vi "pid-waterController.vi"() -> ()   [LabVIEW 2011]
uses:
  <vilib>/Simulation/Scripting/Companion Diagram/SimConfigNode/SimParams.ctl
  <vilib>/Simulation/Scripting/Companion Diagram/SimConfigNode/_simSolvers.ctl
  <vilib>/Simulation/Implementation/Shared/SIMSCR Execution Mode.ctl
  <vilib>/Simulation/Param Hierarchy/Typedefs/SIMPH Param Control Actions.ctl
  <vilib>/Simulation/Implementation/Shared/NILVSim_FinalizeModel.vi
  <vilib>/Simulation/Implementation/Shared/NILVSim_Manager.vi
  <vilib>/Simulation/Implementation/Shared/NILVSim_ParamChanged.vi
  <vilib>/MakerHub/LINX/Public/Peripherals/PWM/PWM Set Duty Cycle 1 Chan.vi
  <vilib>/MakerHub/LINX/Public/Utilities/Open Serial.vi
  <vilib>/Simulation/Implementation/Shared/SIM Unbundle Sim Info.vi
  <vilib>/Simulation/Implementation/Shared/NILVSim_GetModelError.vi
  <vilib>/Simulation/Implementation/Shared/SIM Bundle Sim Info.vi
  <vilib>/Simulation/Implementation/Shared/NILVSim_Initialize.vi
  <vilib>/MakerHub/LINX/Public/Peripherals/PWM/PWM Set Duty Cycle N Chans.vi
  <vilib>/Simulation/Implementation/XNodeFramework/SimXNode/SimX.xnode
  <vilib>/Simulation/Model Libraries/PID/SIM PID (Academic).vi
  <vilib>/Simulation/Model Libraries/PID/SIM PID.vi
  <vilib>/Simulation/Scripting/Companion Diagram/SimConfigNode/SimDog.xnode
  <vilib>/MakerHub/LINX/LMH-LINX.lvlib
  <vilib>/Simulation/Implementation/Shared/NI_SIM_Implementation.lvlib
panel:
  out "PID Output":dbl
  out "Tank":dbl(slide) scale=0.0..10.0
  in  "Derivative time [s] (Td)":dbl=1.0
  in  "Integral time [s] (Ti)":dbl=1.0
  in  "Proportional Gain (Kc)":dbl=1.0
  in  "SetPoint":dbl
  out "Altura\nSensor":dbl
  in  "Serial Port":refnum<visa-resource-name>="N/A"
  out "Altura \nda Água":dbl
  in  "stop":bool
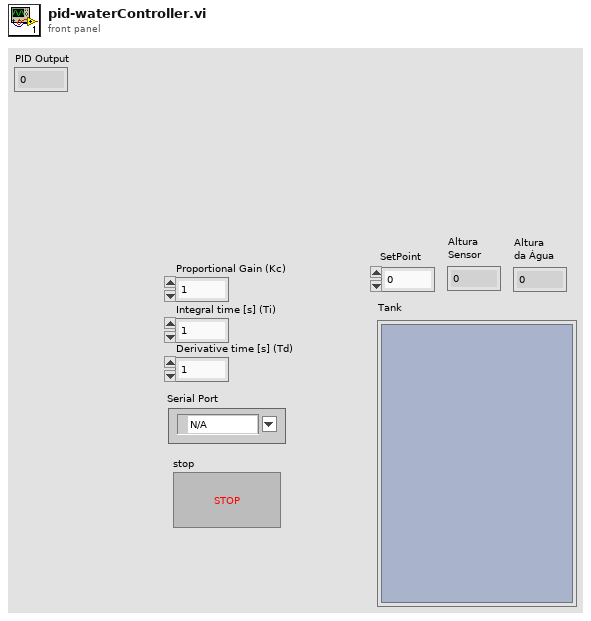
[diagram p1: front panel]
types:
  T1 = typedef "SIMPH Param Control Actions.ctl" = enum16{"get params", "set params"}
  T2 = typedef "SimParams.ctl" = cluster{"Initial Time (s)":dbl, "Final Time (s)":dbl, "Step Size (s)":dbl, "ODE Solver":T3, "Minimum Step Size (s)":dbl, "Maximum Step Size (s)":dbl, "Relative Tolerance":dbl, "Absolute Tolerance":dbl, "Software Timing":bool, "Initial Step Size (s)":dbl, "Automatic Fixed Step Size?":bool, "Automatic Discrete Step Size?":bool, "Discrete Step Size (s)":dbl, "Calculate using Time Step":bool, "Solver Wired?":bool, "Prev.Frm.Expected End":u64, "Prev.Frm.Actual End":u64, "Prev.Frm.Finished Late?":bool, "Prev.Iter.Expected End":u64, "Prev.Iter.Actual End":u64, "Prev.Iter.Finished Late?":bool, "Expected Iteration Start":u64, "Actual Iteration Start":u64, "Expected Frame Start":u64, "Actual Frame Start":u64, "Source Name":string, "Name":string, "Period":i64, "Deadline":i64, "Offset":i64, "Start":i64, "Priority":i32, "Timeout":i32, "Processor":i32, "Mode":enum32{"No Change", "Process missed periods, maintain original phase", "Discard missed periods, maintain original phase", "Process missed periods, ignore original phase", "Discard missed periods, ignore original phase"}, "Wakeup reason":enum32{"Normal", "Aborted", "Asynchronous wakeup", "Timing source error", "Timed loop error", "Timeout"}, "Error":errorcluster, "Source Type":string, "Secondary Source Type":string, "Global End Time":u64, "Global Start Time":u64, "Full Solver Reset":bool, "Execution Mode":T4, "Nan/Inf Check":bool, "Custom Solver Library":string, "Solver Is Variable":bool, "custom solver name":string}
  T3 = typedef "_simSolvers.ctl" = enum16{"Runge-Kutta 1 (Euler)", "Runge-Kutta 2", "Runge-Kutta 3", "Runge-Kutta 4", "Runge-Kutta 23 (variable)", "Runge-Kutta 45 (variable)", "BDF (variable)", "Adams-Moulton (variable)", "Rosenbrock (variable)", "Discrete States Only", "Linearizer", "State Query", "Trim Eval", "Custom Solver"}
  T4 = typedef "SIMSCR Execution Mode.ctl" = u16
  T5 = typedef "LMH-LINX.lvlib/LINX Ref.ctl" = cluster{"IO":T6, "Interface":T7, "LINX Device Config":T8}
  T6 = typedef "LMH-LINX.lvlib/Platform.ctl" = enum16{"Remote", "Local"}
  T7 = typedef "LMH-LINX.lvlib/Interface.ctl" = enum16{"Serial", "TCP"}
  T8 = typedef "LMH-LINX.lvlib/Device.lvlib/LINX Device Config.ctl" = cluster{"Interface":T7, "COM Port":refnum<visa-resource-name>, "TCP Configuration":T9, "Device Family":u8, "Device ID":u8, "Device Name":string, "TCP Ref":refnum<k5>, "Channels":T10}
  T9 = typedef "LMH-LINX.lvlib/Device.lvlib/TCP Config.ctl" = cluster{"IP Address":string, "Port":u16}
  T10 = typedef "LMH-LINX.lvlib/Channels.ctl" = cluster{"DI":u8[], "DO":u8[], "AI":u8[], "AO":u8[], "PWM":u8[], "QE":u8[], "UART":u8[], "I2C 2":u8[], "SPI":u8[], "CAN":u8[], "Servo":u8[], "AI Ref (V)":dbl, "AI Resolution (Bits)":u8, "AO Ref (V)":dbl, "AO Resolution (Bits)":u8}
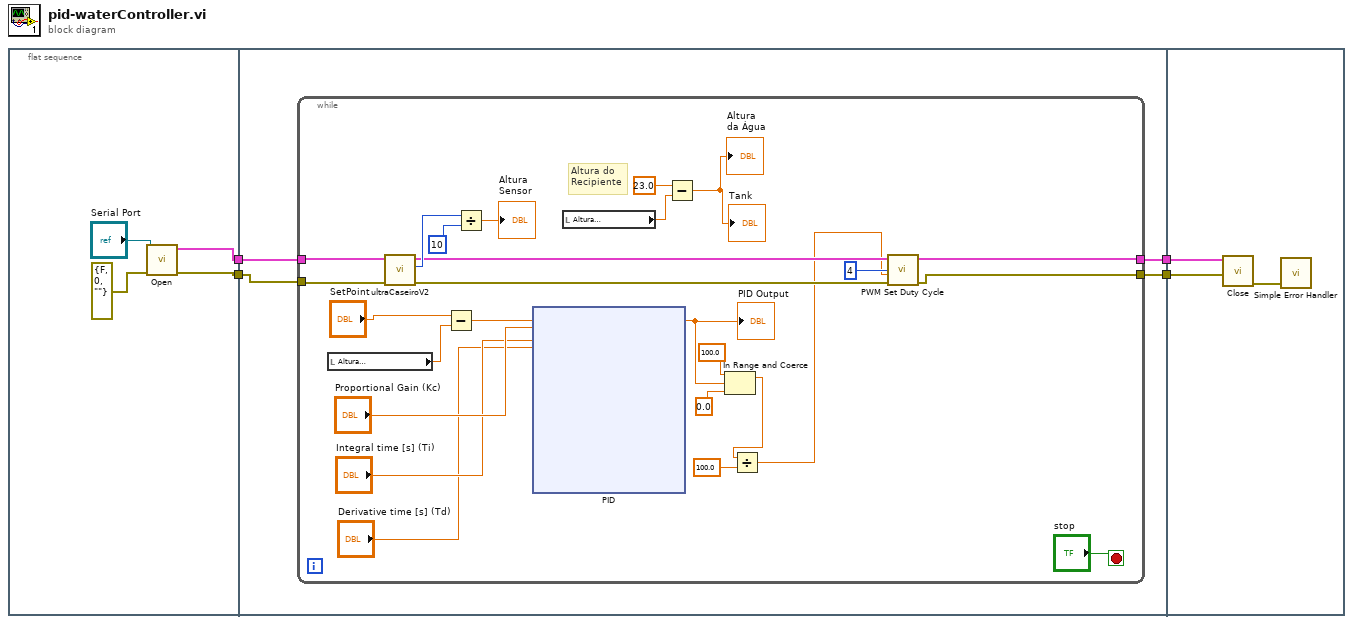
[diagram p0: block diagram]
diagram:
  n1 = flat-sequence {
    tunnel: [w6] -> w4
    tunnel: [w5] -> w3
    tunnel: w4 -> [w12]
    tunnel: w3 -> [w11]
    tunnel: [w10] -> w2
    tunnel: [w9] -> w1
    tunnel: w2 -> [w169]
    tunnel: w1 -> [w168]
    frame #0 {
      n2 = call-poly <vilib>:"Open.vi"("Error In"=errorcluster {"status"=FALSE, "code"=0, "source"=""}, "Serial Port"="Serial Port") -> ("Error Out"=w5:errorcluster, "LINX Resource"=w6:T5)  [unwired: 7 in, 1 out]
    }
    frame #1 {
      n3 = while {
        tunnel: [w20] -> w10
        tunnel: w12 -> [w37]
        tunnel: w11 -> [w36]
        tunnel: [w19] -> w9
        stop <- "stop" stop-if-true
        # "Altura do\nRecipiente"
        n4 = local read "Altura \nda Água"() -> (w28:dbl)
        n5 = call "ultraCaseiroV2.vi"("error in"=w36, "LINX Resource in"=w37) -> ("error out"=w22:errorcluster, "Numeric"=w35:u16, "LINX Resource out"=w23:T5)  [unwired: 7 in]
        n6 = Subtract(x="SetPoint", y=w28) -> (x-y=w30:dbl)
        n7 = Divide(x=w35, y=u16 10) -> (x/y=→"Altura\nSensor":dbl)
        n8 = xnode "PID"("Error"=w30, "Proportional Gain (Kc)"="Proportional Gain (Kc)", "Integral time [s] (Ti)"="Integral time [s] (Ti)", "Derivative time [s] (Td)"="Derivative time [s] (Td)") -> ("Output"=w16:dbl)  [unwired: 2 in, 11 out]
        "PID Output" <- w16
        n9 = local read "Altura\nSensor"() -> (w32:dbl)
        n10 = Subtract(x=23.0, y=w32) -> (x-y=→"Altura \nda Água" →"Tank":dbl)
        n11 = In Range and Coerce(upper limit=100.0, x=w16, lower limit=0.0) -> (coerced(x)=w15:dbl)  [unwired: 1 out]
        n12 = Divide(x=w15, y=100.0) -> (x/y=w13:dbl)
        n13 = call-poly <vilib>:"PWM Set Duty Cycle.vi"("Error In"=w22, "Duty Cycle (0-1)"=w13, "PWM Channel"=u8 4, "LINX Resource"=w23) -> ("Error Out"=w19:errorcluster, "LINX Resource"=w20:T5)  [unwired: 6 in]
      }
    }
    frame #2 {
      n14 = call <vilib>:"Close.vi"("Error In"=w168, "LINX Resource"=w169) -> ("Error Out"=w167:errorcluster)  [unwired: 9 in]
      n15 = call <vilib>:"Simple Error Handler.vi"("error in (no error)"=w167) -> ()  [unwired: 4 in, 5 out]
    }
  }
